vi "Skip Character.vi"(7 "Max Characters":i32=-1, 9 "Stop Strings":string[](array[string]), 10 "Start Index":u32, 11 "JSON":string) -> (0 "Found String Index":i32, 1 "Found Stop Character":bool, 2 "End Index":u32)   [LabVIEW 2011]
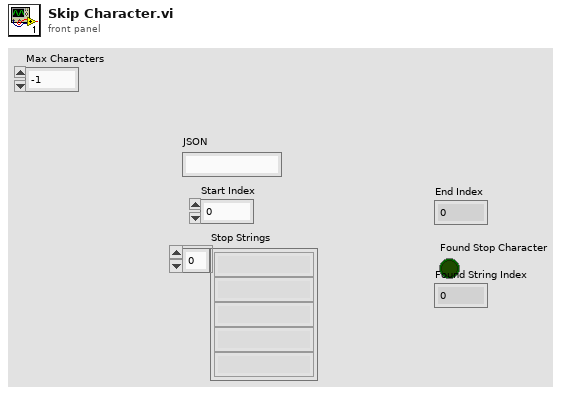
[diagram p1: front panel]
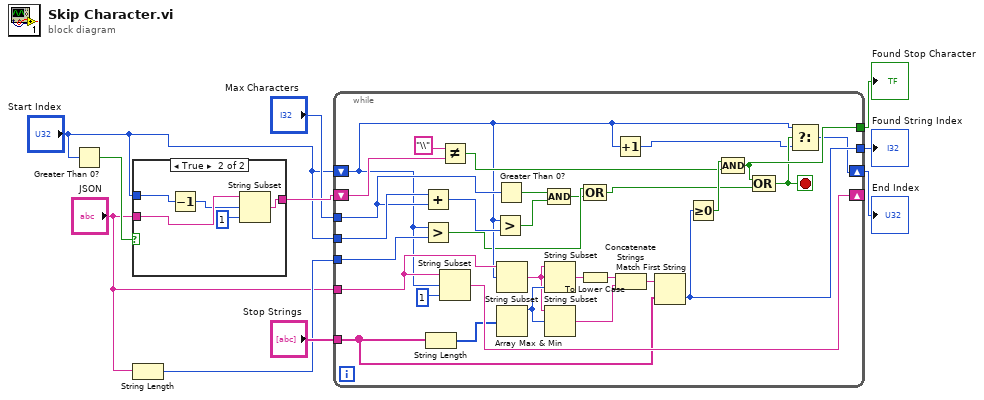
[diagram p0: block diagram]
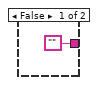
[diagram p2: hidden frame]
diagram:
  n1 = Greater Than 0?(x="Start Index") -> (x > 0?=w5:bool)
  n2 = case shown="True" w5 {
    tunnel: "JSON" -> [_ w16]
    tunnel: "Start Index" -> [_ w15]
    tunnel: ["" ("JSON") w12] -> w3
    frame False {
    }
    frame True {
      n3 = Decrement(x=w15) -> (x-1=w14:u32)
      n4 = String Subset(string=w16, offset (0)=w14, length (rest)=1 ("length (rest)")) -> (substring=w12:string)
    }
  }
  n5 = String Length(string="JSON") -> (length=w9:i32)
  n6 = while {
    tunnel: "JSON" -> [w32]
    shift-right: [w26] -> w8
    shift-left: "Start Index" -> [w20]
    tunnel: w9 -> [w46]
    shift-right: [w45] -> _
    shift-left: w3 -> [w43]
    tunnel: "Stop Strings" -> [w31]
    tunnel: [w30] -> w7
    tunnel: [w29] -> w6
    tunnel: "Max Characters" -> [w24]
    tunnel: "Start Index" -> [w25]
    stop <- w28 stop-if-true
    n7 = Add(x=w25, y=w24) -> (x+y=w21:u32)
    n8 = Greater?(x=w20, y=w46) -> (0:w19:bool)
    n9 = String Length(string=w31) -> (length=w39:i32[])
    n10 = Not Equal?(x="\\", y=w43) -> (x != y?=w40:bool)
    n11 = String Subset(string=w32, offset (0)=w20, length (rest)=1 ("length (rest)")) -> (substring=w45:string)
    n12 = Greater?(x=w20, y=w21) -> (0:w22:bool)
    n13 = Greater Than 0?(x=w24) -> (x > 0?=w23:bool)
    n14 = String Subset(string=w32, offset (0)=w20) -> (substring=w37:string)  [unwired: 1 in]
    n15 = Array Max & Min(array=w39) -> (max value=w38:i32)  [unwired: 3 out]
    n16 = String Subset(string=w37, length (rest)=w38) -> (substring=w36:string)  [unwired: 1 in]
    n17 = String Subset(string=w37, offset (0)=w38) -> (substring=w34:string)  [unwired: 1 in]
    n18 = Compound Arithmetic op=AND(w23, w22) -> (w18:bool)
    n19 = To Lower Case(string=w36) -> (all lower case string=w35:string)
    n20 = Compound Arithmetic op=OR(w19, w18) -> (w17:bool)
    n21 = Increment(x=w20) -> (x+1=w27:u32)
    n22 = Concatenate Strings(w35, w34) -> (w33:string)
    n23 = Match First String(2:w31, 3:w33) -> (0:w29:i32)  [unwired: 1 out]
    n24 = Greater Or Equal To 0?(x=w29) -> (x >= 0?=w41:bool)
    n25 = Compound Arithmetic op=AND(w41, w40) -> (w30:bool)
    n26 = Compound Arithmetic op=OR(w30, w17) -> (w28:bool)
    n27 = Select(t=w20, s=w28, f=w27) -> (s? t:f=w26:u32)
  }
  "End Index" <- w8
  "Found Stop Character" <- w7
  "Found String Index" <- w6
